vi "Add Changed data.vi"(5 "Send any changes now? (F)":bool, 6 "Data changed?":bool, 7 "Data type":T1=enum."Permission level", 8 "error in (no error)":errorcluster, 11 "Fiber Auto Collimation state data in":refnum<class "Fiber Auto Collimation state data.lvclass">) -> (0 "error out":errorcluster, 3 "Fiber Auto Collimation state data out":refnum<class "Fiber Auto Collimation state data.lvclass">)   [LabVIEW 2018, in "Fiber Auto Collimation state data.lvclass"]
doc: "This VI needs to be in all \"Write\" accessors that are part of the State Data class.\n\nThe intent is to automate change tracking so that changes to state data can be easily propogated to the Model loop without undue effort."
uses:
  Fiber Auto Collimation state data.lvclass
  Tracked state data.ctl
  Fiber Auto Collimation state data.lvclass/Fiber Auto Collimation state data.ctl
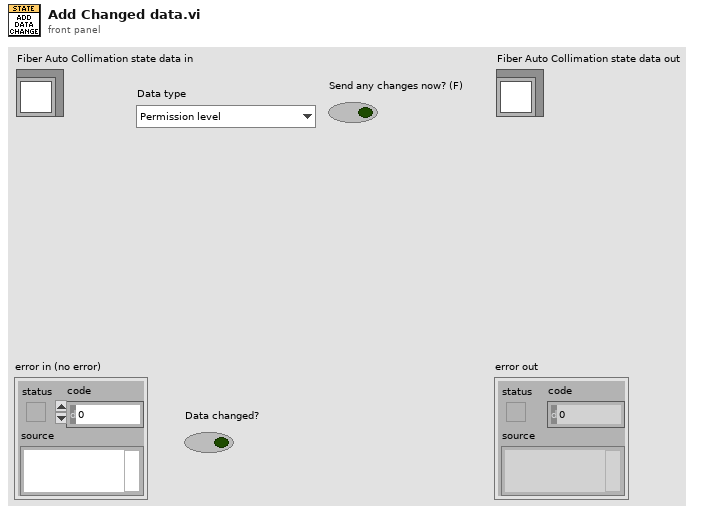
[diagram p1: front panel]
types:
  T1 = typedef "Fiber Auto Collimation state data.lvclass/Tracked state data.ctl" = enum16{"No update", "Permission level", "Username", "Test running", "DUT Serial", "Test status", "MOM Lot", "Loaded test recipe", "Model case running", "Station status", "BV data", "Defect Identify data", "Axis Position data", "Fiber Ass PN", "Operator", "RunTime", "VBAI", "Steps Cycle Time"}
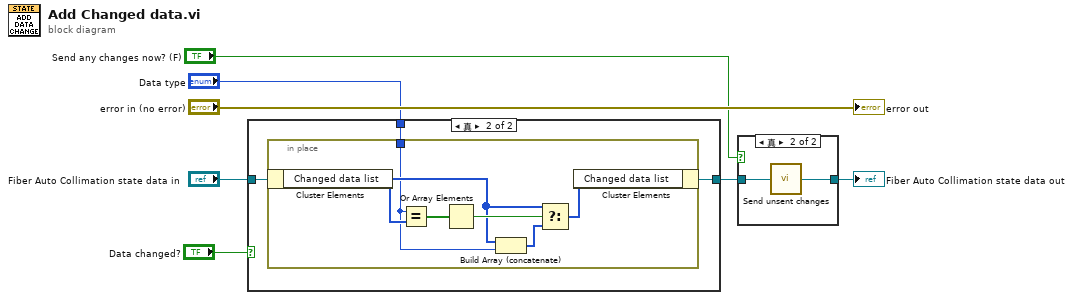
[diagram p0: block diagram]
diagram:
  n1 = case shown="真" "Data changed?" {
    tunnel: "Fiber Auto Collimation state data in" -> [w8 w11]
    tunnel: "Data type" -> [_ w10]
    tunnel: [w8 w9] -> w2
    frame False {
    }
    frame True {
      n2 = in-place {
        in-place-border: w10 -> [w13]
        n3 = in-place-cluster #1(w11) -> ("Changed data list"=w14:T1[])
        n4 = Equal?(x=w13, y=w14) -> (x = y?=w17:bool[])
        n5 = Or Array Elements(Boolean array=w17) -> (logical OR=w16:bool)
        n6 = Build Array (concatenate)(w14, w13) -> (w12:T1[])
        n7 = Select(t=w14, s=w16, f=w12) -> (s? t:f=w15:T1[])
        n8 = in-place-cluster #1("Changed data list"=w15) -> (w9:refnum<class "Fiber Auto Collimation state data.lvclass">)
      }
    }
  }
  n9 = case shown="真" "Send any changes now? (F)" {
    tunnel: w2 -> [w18 w20]
    tunnel: [w18 w19] -> w1
    frame False {
    }
    frame True {
      n10 = call "Send unsent changes.vi"("Fiber Auto Collimation state data in"=w20) -> ("Fiber Auto Collimation state data out"=w19:refnum<class "Fiber Auto Collimation state data.lvclass">)  [unwired: 1 in]
    }
  }
  "Fiber Auto Collimation state data out" <- w1
  "error out" <- "error in (no error)"
